vi "UtilsStr_DeleteEmptyLines.vi"(3 "Input":string[](array[string])) -> (1 "Output":string[](array[string]))   [LabVIEW 2013]
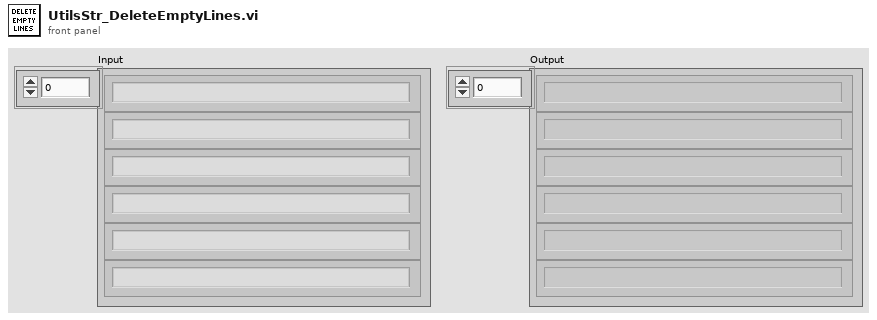
[diagram p1: front panel]
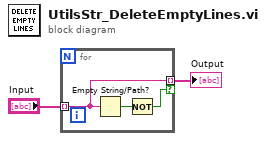
[diagram p0: block diagram]
diagram:
  n1 = for {
    tunnel: "Input" -> [w5] mode=indexing
    tunnel: [w5] -> w1 mode=indexing if=w3
    n2 = Empty String/Path?(string/path=w5) -> (empty?=w4:bool)
    n3 = Not(x=w4) -> (.not. x?=w3:bool)
  }
  "Output" <- w1
